vi "Derivative.vi"(11 "Graph in":cluster{dbl[], dbl[]}) -> (3 "Graph out":cluster{dbl[], "dX/dt":dbl[]})   [LabVIEW 2019]
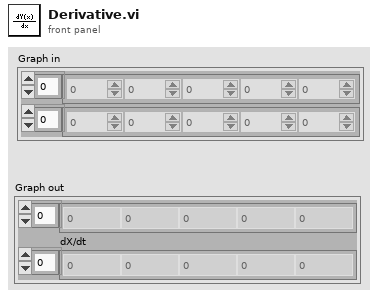
[diagram p1: front panel]
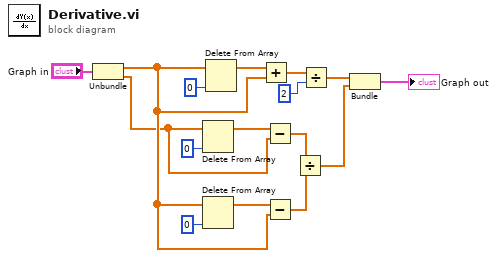
[diagram p0: block diagram]
diagram:
  n1 = Unbundle("Graph in") -> (w2:dbl[], w1:dbl[])
  n2 = Delete From Array(array=w1, index=0) -> (array with subset deleted=w11:dbl[])  [unwired: 1 in, 1 out]
  n3 = Delete From Array(array=w2, index=0) -> (array with subset deleted=w10:dbl[])  [unwired: 1 in, 1 out]
  n4 = Delete From Array(array=w2, index=0) -> (array with subset deleted=w14:dbl[])  [unwired: 1 in, 1 out]
  n5 = Add(x=w14, y=w2) -> (x+y=w15:dbl[])
  n6 = Subtract(x=w11, y=w1) -> (x-y=w8:dbl[])
  n7 = Subtract(x=w10, y=w2) -> (x-y=w7:dbl[])
  n8 = Divide(x=w8, y=w7) -> (x/y=w6:dbl[])
  n9 = Divide(x=w15, y=2 ("mean")) -> (x/y=w5:dbl[])
  n10 = Bundle(w5, w6) -> (→"Graph out":cluster{dbl[], dbl[]})  [unwired: 1 in]
